vi "Operation Window.vi"(6 "Main UI Message Queue":refnum<queue>, 7 "UI State":T2, 8 "error in (no error)":errorcluster, 9 "Graph Notifier":refnum<notifier>, 10 "Message Queues":T21, 11 "Feed Module State Cluster in":T3={"Shared Variables"={"PID 1 Process Variable"="PID1-Mettler Toledo Scale 1", "PID 1 Output"="PID1-Mettler Toledo Scale 1", "PID 1 Setpoint"="PID1-Setpoint", "PID 1 Setpoint SV refnum"="ni.var.psp://localhost/Flow Module 1/PID1-Setpoint", "PID 1 Process Variable SV refnum"="ni.var.psp://localhost/Flow Module 1/PID1-Setpoint", "PID 1 Output SV refnum"="ni.var.psp://localhost/Flow Module 1/PID1-Setpoint"}, "Feed Module Config"={"GUID"="", "Drop Coords"={"Horizontal"=0, "Vertical"=0}, "Process Name"="", "Settings"={"Cycle Period"=500.0, "Ismatech"={"VISA resource name"="", "Simulated?"=TRUE, "Pump Number"=1.0, "Reverse?"=FALSE}, "Masterflex"={"VISA resource name"="", "Simulated?"=TRUE, "Pump Number"=1.0, "Reverse?"=FALSE}, "Mettler"={"VISA resource name"="", "Simulated?"=FALSE}, "Bronkhorst M13 Flow Meter"={"VISA resource name"="", "Simulated?"=TRUE}, "PID 2 Parameters"={"Input Device"=enum."Default", "Output Device"=enum."Default", "Setpoint"=0.0, "PID gains"={"proportional gain (Kc)"=1.0, "integral time (Ti, min)"=0.01, "derivative time (Td, min)"=0.0}}, "Manual Entry"=0.0, "Auto?"=TRUE, "output range"={"output high"=100.0, "output low"=0.0}, "Bronkhorst M14"={"VISA resource name"="", "Simulated?"=FALSE}, "Tacmina Settings"={"Analog DAQ Task"="", "Digital DAQ Task"=""}, "KNF SIMDOS Settings"={"VISA resource name"="", "Simulated?"=TRUE}, "ASIA Pump C"={"ASIA Pump #"=0, "channel"=0, "Simulated"=FALSE}, "VICI Settings"={"VISA resource name"="", "Simulated?"=TRUE, "Pump Letter"="", "Reverse?"=FALSE}, "FLOM Settings"={"VISA resource name"="", "Simulated?"=TRUE, "Pump Number"=0.0}, "SSI PR Settings"={"VISA resource name"="", "Simulated?"=FALSE}}, "Settings Load Count"=0, "OP Load Count"=0}} {"Feed Module Config"."Settings"."output range"."output low" min=0.0 max=100.0 format="%.2f"; "Feed Module Config"."Settings"."output range"."output high" format="%.2f"; "Feed Module Config"."Settings"."PID 2 Parameters"."PID gains"."derivative time (Td, min)" format="%.3f"; "Feed Module Config"."Settings"."PID 2 Parameters"."PID gains"."integral time (Ti, min)" format="%.3f"; "Feed Module Config"."Settings"."PID 2 Parameters"."PID gains"."proportional gain (Kc)" format="%.3f"; "Feed Module Config"."Settings"."ASIA Pump C"."channel" min=0 max=1 step=1; "Feed Module Config"."Settings"."Ismatech"."Pump Number" min=1.0 max=20.0 step=1.0; "Feed Module Config"."Settings"."Masterflex"."Pump Number" min=1.0 max=20.0 step=1.0}) -> (0 "error out":errorcluster, 2 "Need Update":bool, 3 "Feed Module State Cluster out":T3={"Shared Variables"={"PID 1 Process Variable"="PID1-Mettler Toledo Scale 1", "PID 1 Output"="PID1-Mettler Toledo Scale 1", "PID 1 Setpoint"="PID1-Setpoint", "PID 1 Setpoint SV refnum"="ni.var.psp://localhost/Flow Module 1/PID1-Setpoint", "PID 1 Process Variable SV refnum"="ni.var.psp://localhost/Flow Module 1/PID1-Setpoint", "PID 1 Output SV refnum"="ni.var.psp://localhost/Flow Module 1/PID1-Setpoint"}, "Feed Module Config"={"GUID"="", "Drop Coords"={"Horizontal"=0, "Vertical"=0}, "Process Name"="", "Settings"={"Cycle Period"=500.0, "Ismatech"={"VISA resource name"="", "Simulated?"=TRUE, "Pump Number"=1.0, "Reverse?"=FALSE}, "Masterflex"={"VISA resource name"="", "Simulated?"=TRUE, "Pump Number"=1.0, "Reverse?"=FALSE}, "Mettler"={"VISA resource name"="", "Simulated?"=FALSE}, "Bronkhorst M13 Flow Meter"={"VISA resource name"="", "Simulated?"=TRUE}, "PID 2 Parameters"={"Input Device"=enum."Default", "Output Device"=enum."Default", "Setpoint"=0.0, "PID gains"={"proportional gain (Kc)"=1.0, "integral time (Ti, min)"=0.01, "derivative time (Td, min)"=0.0}}, "Manual Entry"=0.0, "Auto?"=TRUE, "output range"={"output high"=100.0, "output low"=0.0}, "Bronkhorst M14"={"VISA resource name"="", "Simulated?"=FALSE}, "Tacmina Settings"={"Analog DAQ Task"="", "Digital DAQ Task"=""}, "KNF SIMDOS Settings"={"VISA resource name"="", "Simulated?"=TRUE}, "ASIA Pump C"={"ASIA Pump #"=0, "channel"=0, "Simulated"=FALSE}, "VICI Settings"={"VISA resource name"="", "Simulated?"=TRUE, "Pump Letter"="", "Reverse?"=FALSE}, "FLOM Settings"={"VISA resource name"="", "Simulated?"=TRUE, "Pump Number"=0.0}, "SSI PR Settings"={"VISA resource name"="", "Simulated?"=FALSE}}, "Settings Load Count"=0, "OP Load Count"=0}} {"Feed Module Config"."Settings"."output range"."output low" min=0.0 max=100.0 format="%.2f"; "Feed Module Config"."Settings"."output range"."output high" format="%.2f"; "Feed Module Config"."Settings"."PID 2 Parameters"."PID gains"."derivative time (Td, min)" format="%.3f"; "Feed Module Config"."Settings"."PID 2 Parameters"."PID gains"."integral time (Ti, min)" format="%.3f"; "Feed Module Config"."Settings"."PID 2 Parameters"."PID gains"."proportional gain (Kc)" format="%.3f"; "Feed Module Config"."Settings"."ASIA Pump C"."channel" min=0 max=1 step=1; "Feed Module Config"."Settings"."Ismatech"."Pump Number" min=1.0 max=20.0 step=1.0; "Feed Module Config"."Settings"."Masterflex"."Pump Number" min=1.0 max=20.0 step=1.0})   [LabVIEW 2018, in "Feed Module.lvlib"]
uses:
  Feed Module/Feed Module.lvlib
  Feed Module/Controls/Feed Message Queues.ctl
  support/Message Queue/Message Cluster.ctl
  Feed Module/Controls/Feed Module State Cluster.ctl
  Feed Module/Controls/Feed Module Shared Variable Cluster.ctl
  Feed Module/Controls/Feed Module Config Cluster.ctl
  <vilib>/Utility/miscctls.llb/LVPoint32TypeDef.ctl
  Feed Module/Controls/Feed Module Settings Cluster.ctl
  Ismatec ISM 831C/Controls/Ismatech Settings Cluster.ctl
  Masterflex 7550-30/Controls/Settings Cluster.ctl
  Mettler Toledo/Controls/Settings Cluster.ctl
  Bronkhorst M13 Flow Meter/Settings Cluster.ctl
  Measure Instrument/PID 2 Parameters Cluster.ctl
  Measure Instrument/PID Input Enum.ctl
  Measure Instrument/PID 2 Output Enum.ctl
  Tacmina QI/Tacmina QI DAQ Setting.ctl
  KNF Pump/Settings Cluster plus SIMDOS.ctl
  ASIA Pump/Pump Settings.ctl
  VICI M50 Party Mode/Settings Cluster.ctl
  FLOM Pump/Settings Cluster.ctl
  SSI PR Class/SSI PR Settings Cluster.ctl
  controls/UI State.ctl
  Config Module/Controls/OP Window Display.ctl
  support/Message Queue/Enqueue Message (Single).vi
  support/Message Queue/Message Queue.lvlib
  support/Support Library.lvlib
  Settings/Settings Dialog.vi
  Settings/Settings.lvlib
  Ismatec ISM 831C/Ismatec ISM 831C.lvlib
  Masterflex 7550-30/Masterflex 7550-30.lvlib
  Mettler Toledo/Mettler Toledo.lvlib
  Bronkhorst M13 Flow Meter/Bronkhorst M13 Flow Meter.lvlib
  Tacmina QI/Tacmina QI.lvlib
  KNF Pump/KNF SIMDOS.lvlib
  ASIA Pump.lvlib
  VICI M50 Party Mode/VICI M6 M50 Party Mode.lvlib
  FLOM Pump/FLOM Pump.lvlib
  SSI PR Class/SSI PR Pump.lvlib
panel:
  out "Start button status":T1(ring)
  out "Started":bool
  out "Updated":bool
  out "Flow":dbl caption="gm/min" format="%.2f"
  out "Data":waveform(dbl)[](graph)
  in  "Auto?":bool=TRUE
  in  "Manual Entry":dbl step=0.1 format="%#_6f"
  in  "Setpoint":dbl
  in  "Cancel Button":bool
  in  "OK Button":bool
  in  "Start":bool
  in  "Settings":bool
  in  "Stop":bool
  # "Output Instruments"
  # "Input Instruments"
  # "Output Instruments"
  # "Input Instruments"
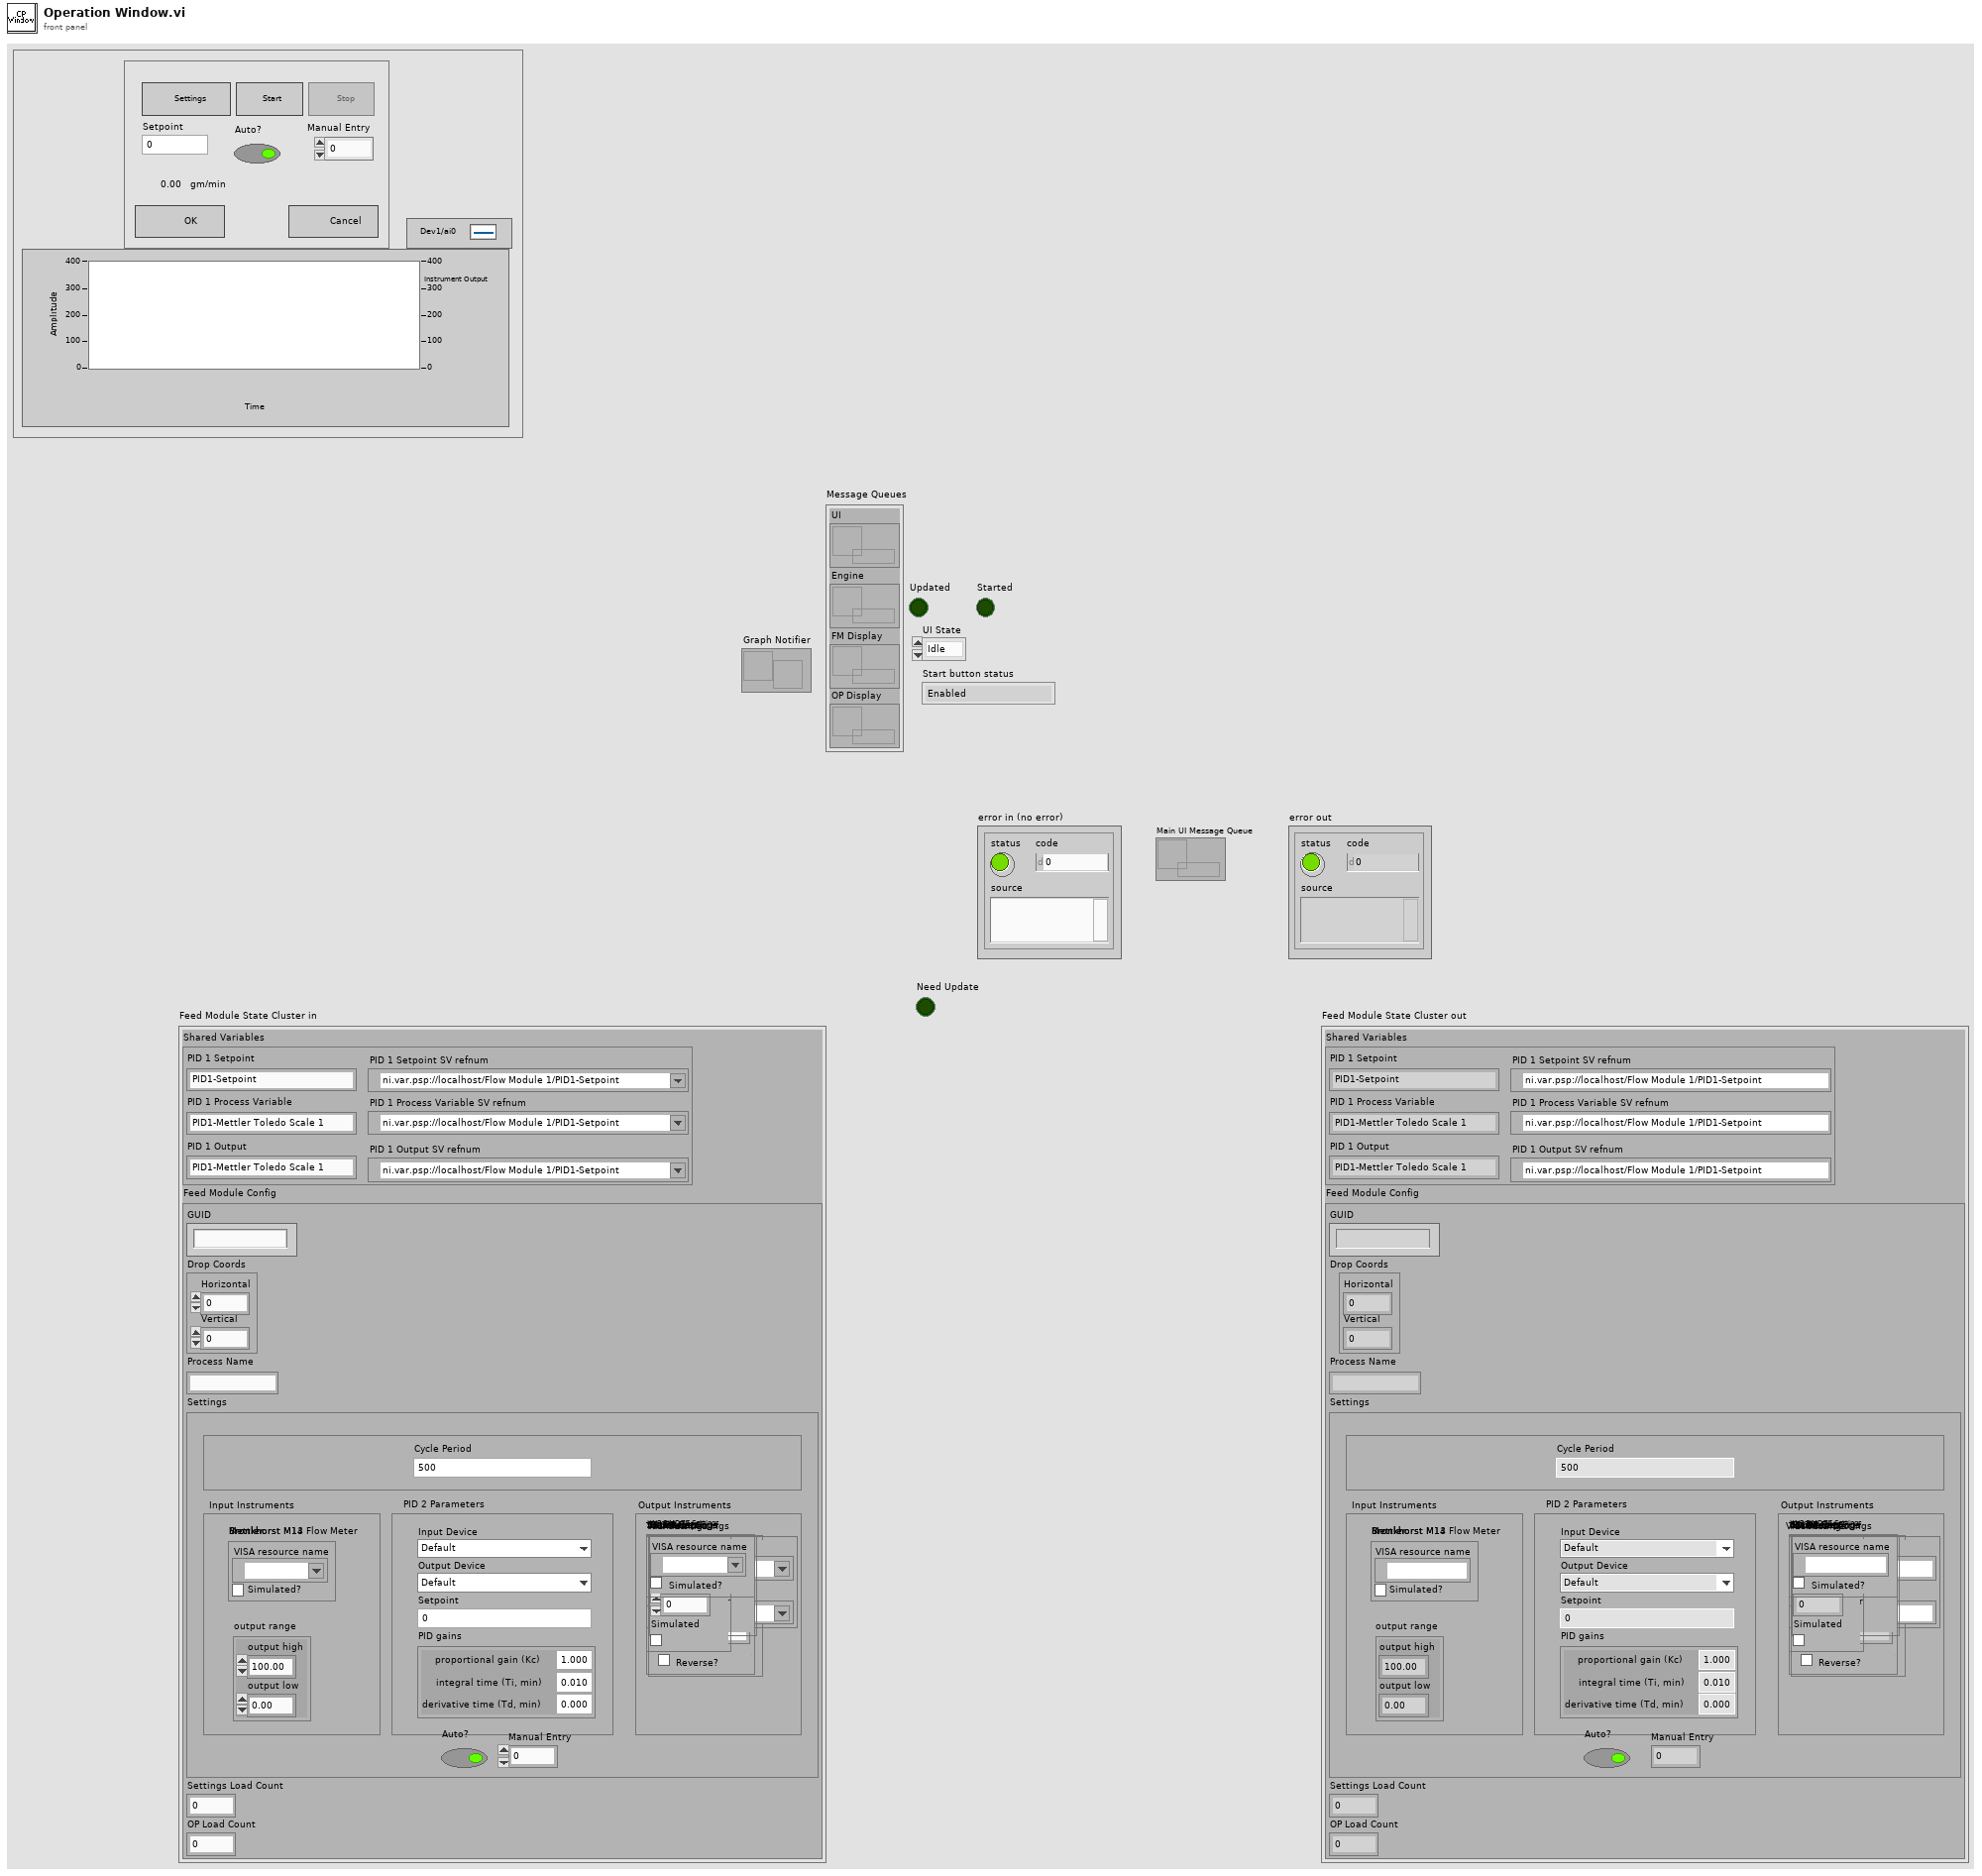
[diagram p1: front panel]
types:
  T1 = enum8{"Enabled", "Disabled", "Disabled and Grayed Out"}
  T2 = typedef "UI State.ctl" = enum16{"Idle", "Acquiring and Logging", "Waiting for Exit", "Waiting for Exit (Acq Stopped)", "Waiting for Exit (Log Stopped)", "Waiting for Stop", "Waiting for Stop (Acq Stopped)", "Waiting for Stop (Log Stopped)"}
  T3 = typedef "Feed Module.lvlib/Feed Module State Cluster.ctl" = cluster{"Shared Variables":T4, "Feed Module Config":T5}
  T4 = typedef "Feed Module.lvlib/Feed Module Shared Variable Cluster.ctl" = cluster{"PID 1 Process Variable":string, "PID 1 Output":string, "PID 1 Setpoint":string, "PID 1 Setpoint SV refnum":refnum<k21>, "PID 1 Process Variable SV refnum":refnum<k21>, "PID 1 Output SV refnum":refnum<k21>}
  T5 = typedef "Feed Module.lvlib/Feed Module Config Cluster.ctl" = cluster{"GUID":string, "Drop Coords":T6, "Process Name":string, "Settings":T7, "Settings Load Count":i32, "OP Load Count":i32}
  T6 = typedef "LVPoint32TypeDef.ctl" = cluster{"Horizontal":i32, "Vertical":i32}
  T7 = typedef "Feed Module.lvlib/Feed Module Settings Cluster.ctl" = cluster{"Cycle Period":dbl, "Ismatech":T8, "Masterflex":T9, "Mettler":T10, "Bronkhorst M13 Flow Meter":T11, "PID 2 Parameters":T12, "Manual Entry":dbl, "Auto?":bool, "output range":cluster{"output high":dbl, "output low":dbl}, "Bronkhorst M14":T10, "Tacmina Settings":T15, "KNF SIMDOS Settings":T16, "ASIA Pump C":T17, "VICI Settings":T18, "FLOM Settings":T19, "SSI PR Settings":T20}
  T8 = typedef "Ismatec ISM 831C.lvlib/Ismatech Settings Cluster.ctl" = cluster{"VISA resource name":refnum<visa-resource-name>, "Simulated?":bool, "Pump Number":dbl, "Reverse?":bool}
  T9 = typedef "Masterflex 7550-30.lvlib/Settings Cluster.ctl" = cluster{"VISA resource name":refnum<visa-resource-name>, "Simulated?":bool, "Pump Number":dbl, "Reverse?":bool}
  T10 = typedef "Mettler Toledo.lvlib/Settings Cluster.ctl" = cluster{"VISA resource name":refnum<visa-resource-name>, "Simulated?":bool}
  T11 = typedef "Bronkhorst M13 Flow Meter.lvlib/Settings Cluster.ctl" = cluster{"VISA resource name":refnum<visa-resource-name>, "Simulated?":bool}
  T12 = typedef "PID 2 Parameters Cluster.ctl" = cluster{"Input Device":T13, "Output Device":T14, "Setpoint":dbl, "PID gains":cluster{"proportional gain (Kc)":dbl, "integral time (Ti, min)":dbl, "derivative time (Td, min)":dbl}}
  T13 = typedef "PID Input Enum.ctl" = enum16{"Default", "Bronkhorst M13", "Bronkhorst M14", "Scale Rate of Change"}
  T14 = typedef "PID 2 Output Enum.ctl" = enum16{"Default", "Ismatec ISM 831C", "Masterflex 7550-30", "VICI", "Tacmina QI", "KNF SIMDOS", "ASIA Type C", "FLOM UI-22-11", "SSI PR"}
  T15 = typedef "Tacmina QI.lvlib/Tacmina QI DAQ Setting.ctl" = cluster{"Analog DAQ Task":refnum<k21>, "Digital DAQ Task":refnum<k21>}
  T16 = typedef "KNF SIMDOS.lvlib/Settings Cluster plus SIMDOS.ctl" = cluster{"VISA resource name":refnum<visa-resource-name>, "Simulated?":bool}
  T17 = typedef "ASIA Pump.lvlib/Pump Settings.ctl" = cluster{"ASIA Pump #":i32, "channel":i32, "Simulated":bool}
  T18 = typedef "VICI M6 M50 Party Mode.lvlib/Settings Cluster.ctl" = cluster{"VISA resource name":refnum<visa-resource-name>, "Simulated?":bool, "Pump Letter":string, "Reverse?":bool}
  T19 = typedef "FLOM Pump.lvlib/Settings Cluster.ctl" = cluster{"VISA resource name":refnum<visa-resource-name>, "Simulated?":bool, "Pump Number":dbl}
  T20 = typedef "SSI PR Pump.lvlib/SSI PR Settings Cluster.ctl" = cluster{"VISA resource name":refnum<visa-resource-name>, "Simulated?":bool}
  T21 = typedef "Feed Module.lvlib/Feed Message Queues.ctl" = cluster{"UI":refnum<queue>, "Engine":refnum<queue>, "FM Display":refnum<queue>, "OP Display":refnum<queue>}
  T22 = typedef "Feed Module.lvlib/OP Window Display.ctl" = cluster{"Flow":dbl, "Manual":dbl, "Pump Status":u16}
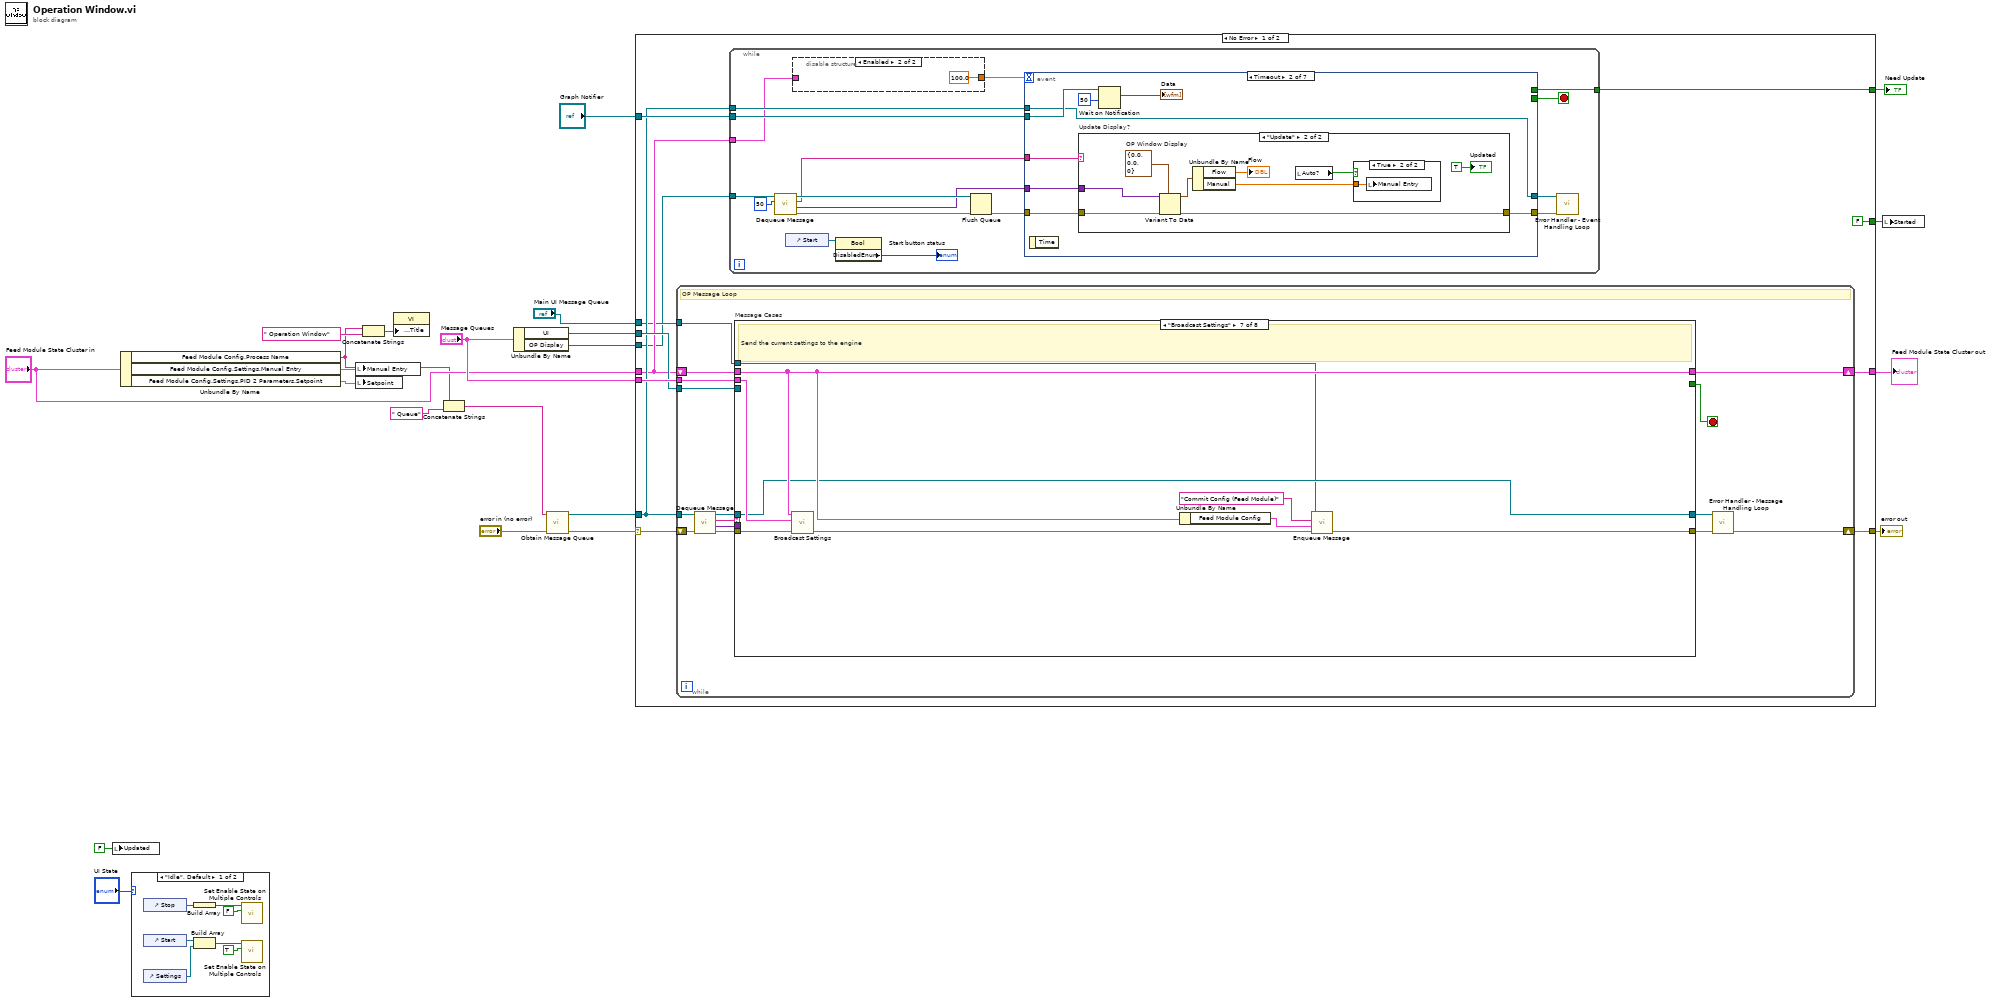
[diagram p0: block diagram]
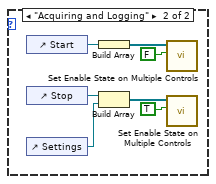
[diagram p2: hidden frame]
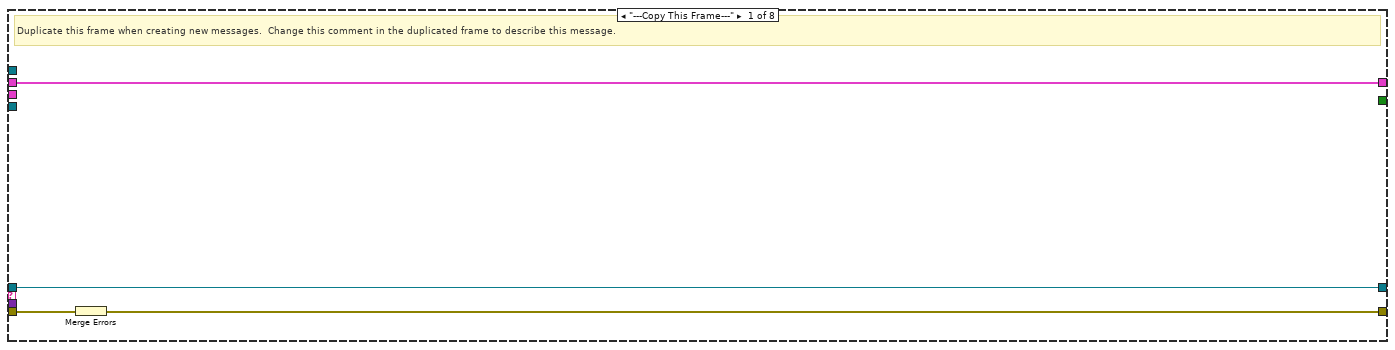
[diagram p3: hidden frame]
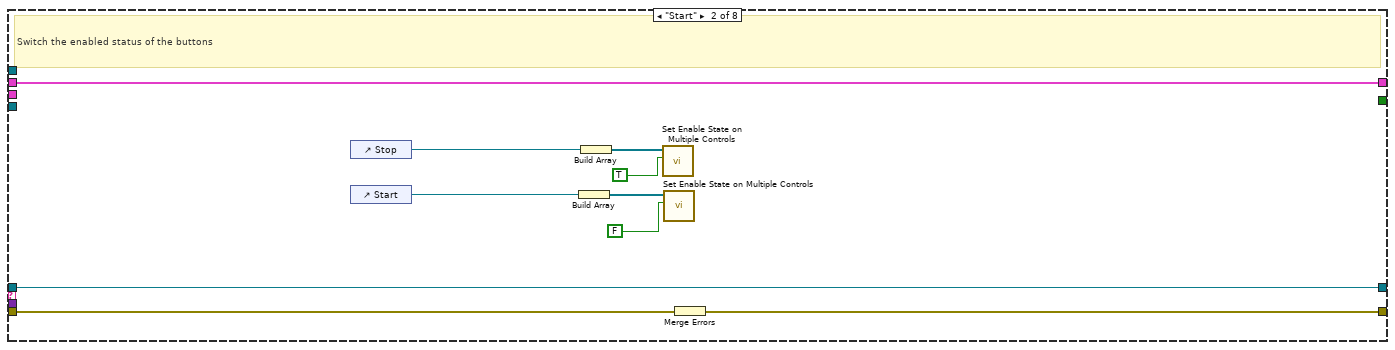
[diagram p4: hidden frame]
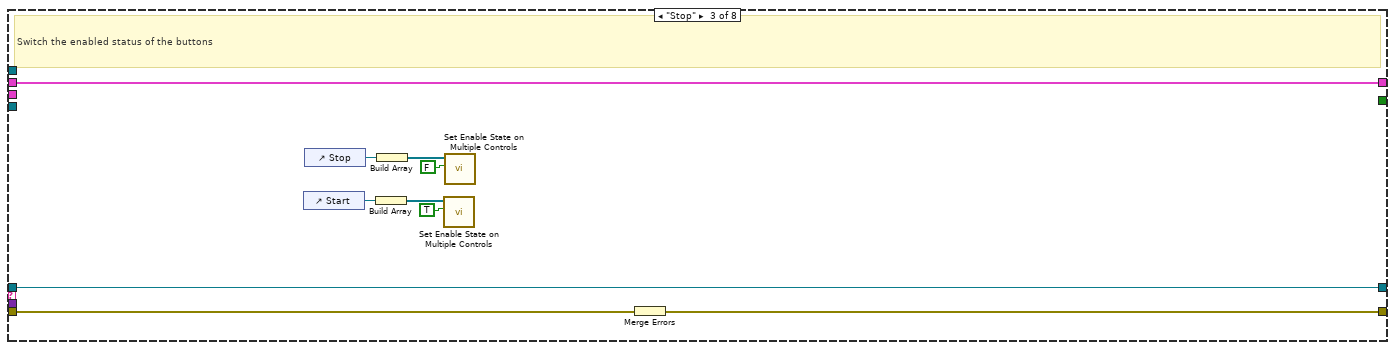
[diagram p5: hidden frame]
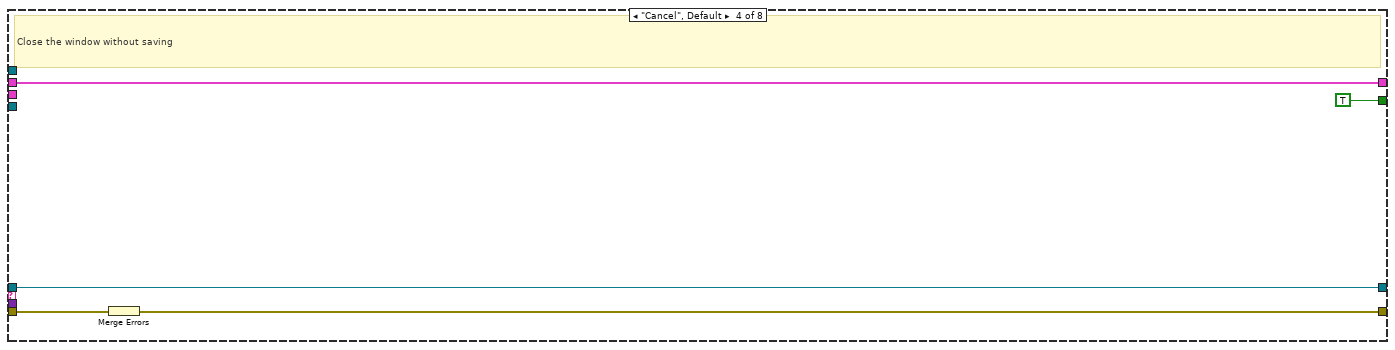
[diagram p6: hidden frame]
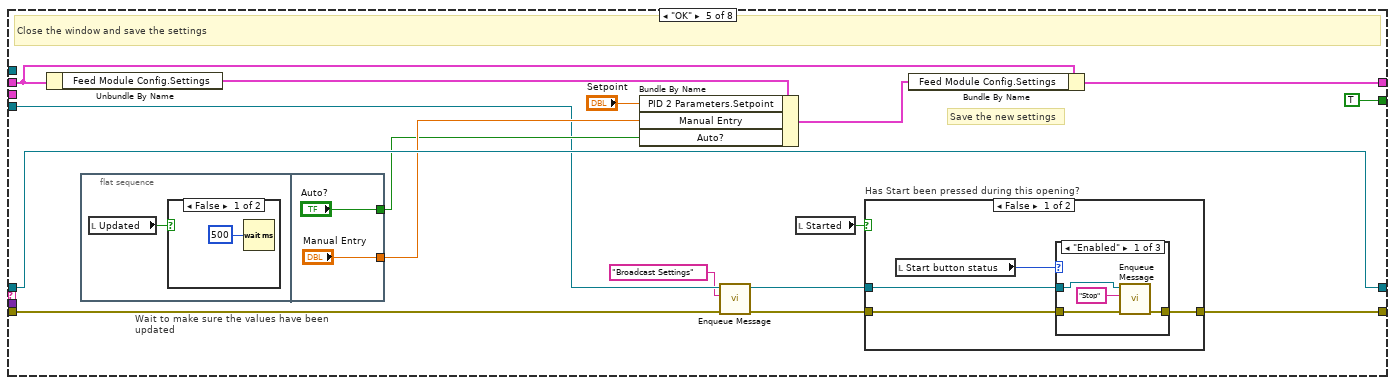
[diagram p7: hidden frame]
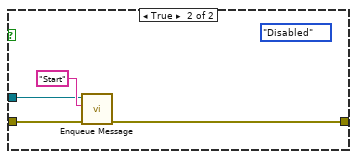
[diagram p10: hidden frame]
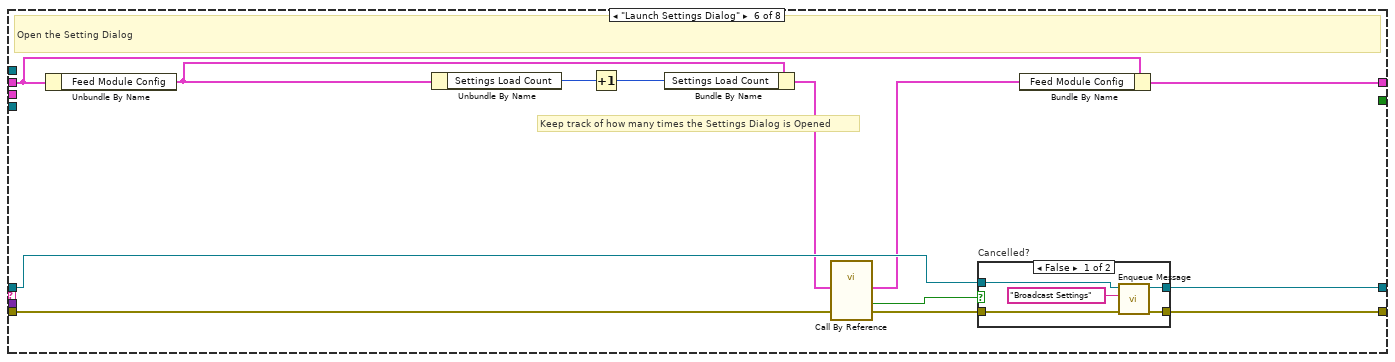
[diagram p12: hidden frame]
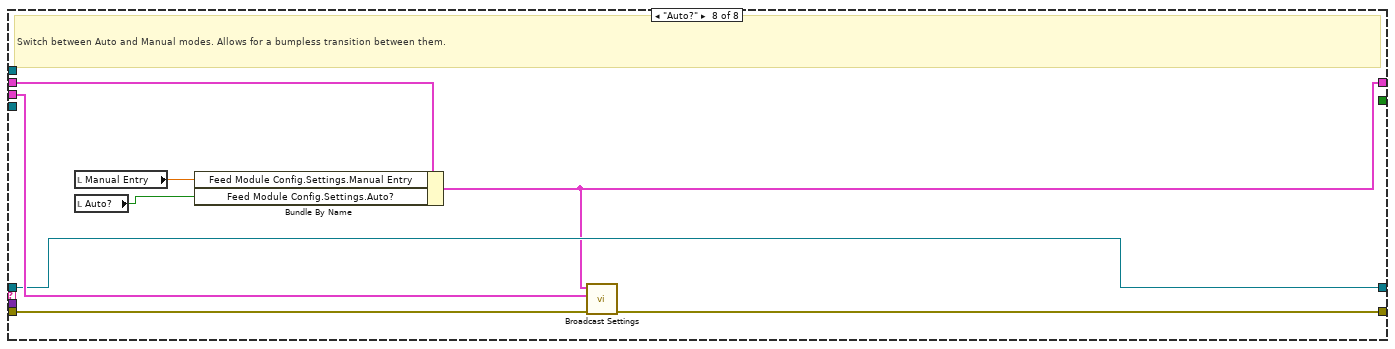
[diagram p14: hidden frame]
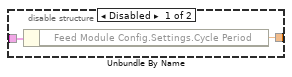
[diagram p15: hidden frame]
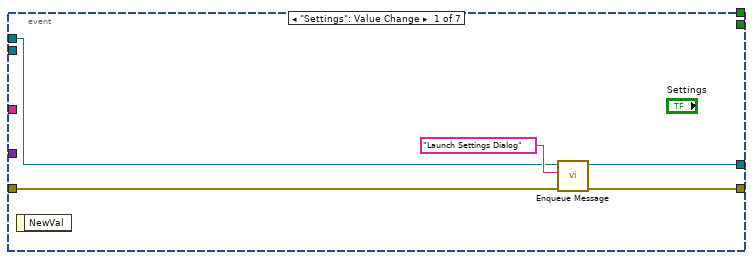
[diagram p16: hidden frame]
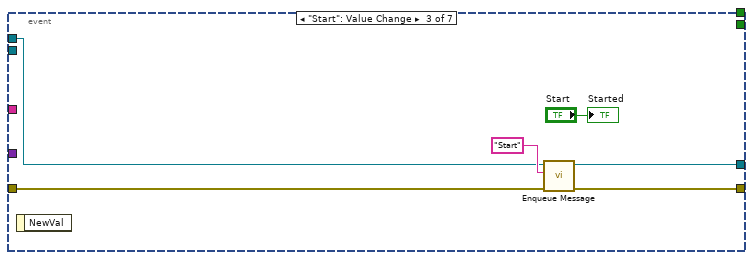
[diagram p19: hidden frame]
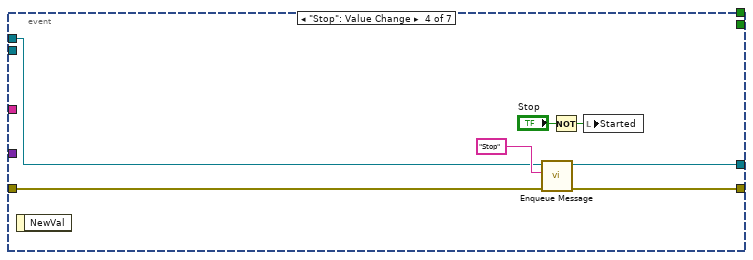
[diagram p20: hidden frame]
diagram:
  n1 = local write "Updated"(FALSE ("Boolean")) -> ()
  n2 = Unbundle By Name("Feed Module State Cluster in") -> ("Feed Module Config.Process Name"=w6:string, "Feed Module Config.Settings.Manual Entry"=w12:dbl, "Feed Module Config.Settings.PID 2 Parameters.Setpoint"=w10:dbl)
  n3 = case shown="\"Idle\", Default" "UI State" {
    frame "Idle", Default {
      n4 = control-ref of="Stop"() -> (w23:refnum<vi>)
      n5 = control-ref of="Start"() -> (w25:refnum<vi>)
      n6 = control-ref of="Settings"() -> (w24:refnum<vi>)
      n7 = Build Array(w23) -> (w27:refnum<vi>[])
      n8 = Build Array(w25, w24) -> (w28:refnum<vi>[])
      n9 = call "Set Enable State on Multiple Controls.vi"("Enable?"=FALSE, "Controls"=w27) -> ()  [unwired: 10 in]
      n10 = call "Set Enable State on Multiple Controls.vi"("Enable?"=TRUE, "Controls"=w28) -> ()  [unwired: 10 in]
    }
    frame "Acquiring and Logging" {
      n11 = control-ref of="Start"() -> (w32:refnum<vi>)
      n12 = control-ref of="Stop"() -> (w31:refnum<vi>)
      n13 = control-ref of="Settings"() -> (w30:refnum<vi>)
      n14 = Build Array(w32) -> (w35:refnum<vi>[])
      n15 = Build Array(w31, w30) -> (w34:refnum<vi>[])
      n16 = call "Set Enable State on Multiple Controls.vi"("Enable?"=FALSE, "Controls"=w35) -> ()  [unwired: 10 in]
      n17 = call "Set Enable State on Multiple Controls.vi"("Enable?"=TRUE, "Controls"=w34) -> ()  [unwired: 10 in]
    }
  }
  n18 = local write "Manual Entry"(w12) -> ()
  n19 = local write "Setpoint"(w10) -> ()
  n20 = Concatenate Strings(w6, " Operation Window" ("string")) -> (w5:string)
  n21 = property class="VI"("Front Panel.Title"=w5) -> ()  [unwired: 2 in, 2 out]
  n22 = Concatenate Strings(w6, " Queue" ("string")) -> (w9:string)
  n23 = Unbundle By Name("Message Queues") -> ("UI"=w16:refnum<queue>, "OP Display"=w13:refnum<queue>)
  n24 = call "Obtain Message Queue.vi"("error in (no error)"="error in (no error)", "name (unnamed)"=w9) -> ("error out"=w2:errorcluster, "Message Queue"=w19:refnum<queue>)  [unwired: 8 in]
  n25 = case shown="No Error" w2 {
    selector: w2 -> [w37 w243]
    tunnel: [w41 w243] -> w22
    tunnel: [w48 FALSE] -> w21
    tunnel: w19 -> [w43 _]
    tunnel: "Feed Module State Cluster in" -> [w42 w241]
    tunnel: [w47 w241] -> w14
    tunnel: "Message Queues" -> [w46 _]
    tunnel: "Graph Notifier" -> [w45 _]
    tunnel: w16 -> [w44 _]
    tunnel: "Main UI Message Queue" -> [w40 _]
    tunnel: w13 -> [w39 _]
    tunnel: [FALSE FALSE] -> w3
    frame No Error {
      n26 = while {
        shift-right: [w52] -> w41
        shift-left: w37 -> [w55]
        tunnel: w43 -> [w54]
        tunnel: w46 -> [w56]
        shift-right: [w57] -> w47
        shift-left: w42 -> [w53]
        tunnel: w44 -> [w51]
        tunnel: w40 -> [w49]
        stop <- w58 stop-if-true
        # "OP Message Loop"
        n27 = call "Dequeue Message.vi"("error in (no error)"=w55, "Message Queue"=w54) -> ("error out"=w59:errorcluster, "Message Data"=w62:variant, "Message"=w63:string, "dup Message Queue"=w60:refnum<queue>)  [unwired: 6 in]
        n28 = case "Message Cases" shown="\"Broadcast Settings\"" w63 {
          tunnel: w60 -> [w64 w68 w78 w88 w106 w135 w152 w161]
          tunnel: w59 -> [w67 w77 w87 w92 w98 w128 w154 w162]
          tunnel: [w66 w76 w86 w91 w96 w137 w151 w156] -> w61
          tunnel: w62 -> [_ _ _ _ _ _ _ _]
          tunnel: [_ _ _ TRUE TRUE _ _ _] -> w58
          tunnel: w53 -> [w65 w69 w85 w89 w102 w136 w153 w158]
          tunnel: [w65 w69 w85 w89 w105 w130 w153 w157] -> w57
          tunnel: w56 -> [_ _ _ _ _ _ w155 w163]
          tunnel: w51 -> [_ _ _ _ w99 _ _ _]
          tunnel: [w64 w68 w78 w88 w106 w134 w152 w161] -> w50
          tunnel: w49 -> [_ _ _ _ _ _ w148 _]
          frame "---Copy This Frame---" {
            # "Duplicate this frame when creating new messages.  Change this comment in the duplicated frame to describe this message."
            n29 = Merge Errors(w67) -> (w66:errorcluster)
          }
          frame "Start" {
            # "Switch the enabled status of the buttons"
            n30 = control-ref of="Stop"() -> (w74:refnum<vi>)
            n31 = control-ref of="Start"() -> (w75:refnum<vi>)
            n32 = Build Array(w75) -> (w72:refnum<vi>[])
            n33 = Build Array(w74) -> (w73:refnum<vi>[])
            n34 = call "Set Enable State on Multiple Controls.vi"("Enable?"=TRUE, "Controls"=w73) -> ()  [unwired: 10 in]
            n35 = call "Set Enable State on Multiple Controls.vi"("Enable?"=FALSE, "Controls"=w72) -> ()  [unwired: 10 in]
            n36 = Merge Errors(w77) -> (w76:errorcluster)
          }
          frame "Stop" {
            # "Switch the enabled status of the buttons"
            n37 = control-ref of="Start"() -> (w84:refnum<vi>)
            n38 = control-ref of="Stop"() -> (w81:refnum<vi>)
            n39 = Build Array(w84) -> (w83:refnum<vi>[])
            n40 = Build Array(w81) -> (w80:refnum<vi>[])
            n41 = call "Set Enable State on Multiple Controls.vi"("Enable?"=TRUE, "Controls"=w83) -> ()  [unwired: 10 in]
            n42 = call "Set Enable State on Multiple Controls.vi"("Enable?"=FALSE, "Controls"=w80) -> ()  [unwired: 10 in]
            n43 = Merge Errors(w87) -> (w86:errorcluster)
          }
          frame "Cancel", Default {
            # "Close the window without saving"
            n44 = Merge Errors(w92) -> (w91:errorcluster)
          }
          frame "OK" {
            # "Save the new settings"
            # "Close the window and save the settings"
            n45 = Unbundle By Name(w102) -> ("Feed Module Config.Settings"=w103:T7)
            n46 = flat-sequence "Wait to make sure the values have been updated" {
              tunnel: ["Manual Entry"] -> w101
              tunnel: ["Auto?"] -> w100
              frame #0 {
                n47 = local read "Updated"() -> (w123:bool)
                n48 = case shown="False" w123 {
                  frame False {
                    n49 = Wait (ms)(milliseconds to wait=u32 500) -> ()  [unwired: 1 out]
                  }
                  frame True {
                  }
                }
              }
              frame #1 {
              }
            }
            n50 = Bundle By Name(cluster=w103, "PID 2 Parameters.Setpoint"="Setpoint", "Manual Entry"=w101, "Auto?"=w100) -> (w104:T7)
            n51 = call-poly "Enqueue Message.vi"("error in (no error)"=w98, "Message"="Broadcast Settings", "Message Queue"=w99) -> ("error out"=w93:errorcluster, "dup Message Queue"=w94:refnum<queue>)  [unwired: 7 in]
            n52 = local read "Started"() -> (w97:bool)
            n53 = case "Has Start been pressed during this opening?" shown="False" w97 {
              tunnel: w94 -> [w110 w121]
              tunnel: w93 -> [w111 w120]
              tunnel: [w112 w119] -> w96
              frame False {
                n54 = local read "Start button status"() -> (w109:T1)
                n55 = case shown="\"Enabled\"" w109 {
                  tunnel: [w115 w117 w118] -> w112
                  tunnel: w111 -> [w114 w117 w118]
                  tunnel: w110 -> [w113 _ _]
                  frame "Enabled" {
                    n56 = call-poly "Enqueue Message.vi"("error in (no error)"=w114, "Message"="Stop", "Message Queue"=w113) -> ("error out"=w115:errorcluster)  [unwired: 7 in, 1 out]
                  }
                  frame "Disabled" {
                  }
                  frame "Disabled and Grayed Out" {
                  }
                }
              }
              frame True {
                (unwired) T1."Disabled" ("DisabledEnum")
                n57 = call-poly "Enqueue Message.vi"("error in (no error)"=w120, "Message"="Start", "Message Queue"=w121) -> ("error out"=w119:errorcluster)  [unwired: 7 in, 1 out]
              }
            }
            n58 = Bundle By Name(cluster=w102, "Feed Module Config.Settings"=w104) -> (w105:T3)
          }
          frame "Launch Settings Dialog" {
            # "Keep track of how many times the Settings Dialog is Opened"
            # "Open the Setting Dialog"
            n59 = Unbundle By Name(w136) -> ("Feed Module Config"=w132:T5)
            n60 = Unbundle By Name(w132) -> ("Settings Load Count"=w131:i32)
            n61 = Increment(x=w131) -> (x+1=w133:i32)
            n62 = Bundle By Name(cluster=w132, "Settings Load Count"=w133) -> (w127:T5)
            n63 = call-by-ref "?"("error in (no error)"=w128, "Feed Module Config in"=w127) -> ("error out"=w138:errorcluster, "Cancelled?"=w139:bool, "Feed Module Config out"=w129:T5)  [unwired: 8 in, 3 out]
            n64 = case "Cancelled?" shown="False" w139 {
              tunnel: [w144 w146] -> w137
              tunnel: w138 -> [w142 w146]
              tunnel: w135 -> [w141 w145]
              tunnel: [w140 w145] -> w134
              frame False {
                n65 = call-poly "Enqueue Message.vi"("error in (no error)"=w142, "Message"="Broadcast Settings", "Message Queue"=w141) -> ("error out"=w144:errorcluster, "dup Message Queue"=w140:refnum<queue>)  [unwired: 7 in]
              }
              frame True {
              }
            }
            n66 = Bundle By Name(cluster=w136, "Feed Module Config"=w129) -> (w130:T3)
          }
          frame "Broadcast Settings" {
            # "Send the current settings to the engine"
            n67 = call "Broadcast Settings.vi"("error in (no error)"=w154, "Message Queues"=w155, "Feed Module State Cluster in"=w153) -> ("error out"=w150:errorcluster)  [unwired: 8 in]
            n68 = Unbundle By Name(w153) -> ("Feed Module Config"=w149:T5)
            n69 = call-poly "Enqueue Message.vi"("error in (no error)"=w150, "Message Data"=w149, "Message"="Commit Config (Feed Module)", "Message Queue"=w148) -> ("error out"=w151:errorcluster)  [unwired: 6 in, 1 out]
          }
          frame "Auto?" {
            # "Switch between Auto and Manual modes. Allows for a bumpless transition between them."
            n70 = local read "Manual Entry"() -> (w160:dbl)
            n71 = local read "Auto?"() -> (w159:bool)
            n72 = Bundle By Name(cluster=w158, "Feed Module Config.Settings.Manual Entry"=w160, "Feed Module Config.Settings.Auto?"=w159) -> (w157:T3)
            n73 = call "Broadcast Settings.vi"("error in (no error)"=w162, "Message Queues"=w163, "Feed Module State Cluster in"=w157) -> ("error out"=w156:errorcluster)  [unwired: 8 in]
          }
        }
        n74 = call "Error Handler - Message Handling Loop.vi"("error in (no error)"=w61, "Message Queue"=w50) -> ("dup error in"=w52:errorcluster)  [unwired: 8 in, 1 out]
      }
      n75 = while {
        tunnel: [w177] -> w48
        tunnel: w43 -> [w176]
        tunnel: w45 -> [w175]
        tunnel: w42 -> [w173]
        tunnel: w39 -> [w172]
        stop <- w178 stop-if-true
        n76 = call "Dequeue Message.vi"("timeout in ms (-1)"=50, "Message Queue"=w172) -> ("error out"=w170:errorcluster, "Message Data"=w167:variant, "Message"=w168:string, "dup Message Queue"=w169:refnum<queue>)  [unwired: 6 in]
        n77 = control-ref of="Start"() -> (w165:refnum<vi>)
        n78 = disable-structure shown="Enabled" {
          disable-tunnel: [w182 100.0 ("Cycle Period")] -> w174
          disable-tunnel: w173 -> [w181 _]
          frame Disabled {
            n79 = Unbundle By Name(w181) -> ("Feed Module Config.Settings.Cycle Period"=w182:dbl)
          }
          frame Enabled {
          }
        }
        n80 = property class="Bool"(reference=w165) -> ("DisabledEnum"=→"Start button status":T1)  [unwired: 1 in, 2 out]
        n81 = Flush Queue(queue=w169, error in (no error)=w170) -> (error out=w166:errorcluster)  [unwired: 2 out]
        n82 = event shown="[1] Timeout" {
          selector: _ -> [_ _ _ _ _ _ _]
          dyn-events: _ -> [_ _ _ _ _ _ _]
          timeout: w174 -> [_ _ _ _ _ _ _]
          tunnel: [w187 w189 w210 w218 w223 w230 w238] -> w180
          tunnel: [w186 w190 w211 w217 w222 w229 w237] -> w179
          tunnel: [_ _ _ _ _ TRUE ("Priority Message? (F)") w236] -> w178
          tunnel: [_ _ _ _ _ FALSE ("Priority Message? (F)") w236] -> w177
          tunnel: w176 -> [w185 w189 w212 w219 w224 w227 w235]
          tunnel: w175 -> [_ w195 _ _ _ _ _]
          tunnel: w168 -> [_ w193 _ _ _ _ _]
          tunnel: w167 -> [_ w192 _ _ _ _ _]
          tunnel: w166 -> [w184 w191 w208 w214 w221 w226 w234]
          event "Settings": Value Change {
            n83 = event-data() -> ()  [unwired: 1 in, 1 out]
            n84 = call-poly "Enqueue Message.vi"("error in (no error)"=w184, "Message"="Launch Settings Dialog", "Message Queue"=w185) -> ("error out"=w186:errorcluster, "dup Message Queue"=w187:refnum<queue>)  [unwired: 7 in]
          }
          event Timeout {
            n85 = event-data() -> ()  [unwired: 1 in, 1 out]
            n86 = case "Update Display?" shown="\"Update\"" w193 {
              tunnel: w192 -> [_ w206]
              tunnel: w191 -> [w197 w199]
              tunnel: [w197 w198] -> w190
              frame "False", Default {
              }
              frame "Update" {
                w205 = T22 {"Flow"=0.0, "Manual"=0.0, "Pump Status"=0}  # OP Window Display
                n87 = Variant To Data(error in=w199, type=w205, Variant=w206) -> (data=w204:T22, error out=w198:errorcluster)
                n88 = Unbundle By Name(w204) -> ("Flow"=→"Flow":dbl, "Manual"=w202:dbl)
                n89 = local read "Auto?"() -> (w201:bool)
                n90 = case shown="True" w201 {
                  tunnel: w202 -> [_ w207]
                  frame False {
                  }
                  frame True {
                    n91 = local write "Manual Entry"(w207) -> ()
                  }
                }
                "Updated" <- TRUE ("Boolean")
              }
            }
            n92 = Wait on Notification(notifier=w195, timeout in ms (-1)=50) -> (notification=→"Data":waveform(dbl)[])  [unwired: 2 in, 3 out]
          }
          event "Start": Value Change {
            n93 = event-data() -> ()  [unwired: 1 in, 1 out]
            n94 = call-poly "Enqueue Message.vi"("error in (no error)"=w208, "Message"="Start", "Message Queue"=w212) -> ("error out"=w211:errorcluster, "dup Message Queue"=w210:refnum<queue>)  [unwired: 7 in]
            "Started" <- "Start"
          }
          event "Stop": Value Change {
            n95 = event-data() -> ()  [unwired: 1 in, 1 out]
            n96 = call-poly "Enqueue Message.vi"("error in (no error)"=w214, "Message"="Stop", "Message Queue"=w219) -> ("error out"=w217:errorcluster, "dup Message Queue"=w218:refnum<queue>)  [unwired: 7 in]
            n97 = Not(x="Stop") -> (.not. x?=w215:bool)
            n98 = local write "Started"(w215) -> ()
          }
          event "Auto?": Value Change {
            n99 = event-data() -> ()  [unwired: 1 in, 1 out]
            n100 = call-poly "Enqueue Message.vi"("error in (no error)"=w221, "Message"="Auto?", "Message Queue"=w224) -> ("error out"=w222:errorcluster, "dup Message Queue"=w223:refnum<queue>)  [unwired: 7 in]
          }
          event "Cancel Button": Value Change {
            n101 = event-data() -> ()  [unwired: 1 in, 1 out]
            n102 = call-poly "Enqueue Message.vi"("Priority Message? (F)"=TRUE, "error in (no error)"=w226, "Message"="Cancel", "Message Queue"=w227) -> ("error out"=w229:errorcluster, "dup Message Queue"=w230:refnum<queue>)  [unwired: 6 in]
          }
          event "OK Button": Value Change {
            w236 = TRUE
            n103 = event-data() -> ()  [unwired: 1 in, 1 out]
            n104 = call-poly "Enqueue Message.vi"("error in (no error)"=w234, "Message"="OK", "Message Queue"=w235) -> ("error out"=w237:errorcluster, "dup Message Queue"=w238:refnum<queue>)  [unwired: 7 in]
          }
        }
        n105 = call "Error Handler - Event Handling Loop.vi"("error in (no error)"=w179, "Message Queue"=w180) -> ()  [unwired: 8 in, 2 out]
      }
    }
    frame Error {
    }
  }
  "error out" <- w22
  "Need Update" <- w21
  "Feed Module State Cluster out" <- w14
  n106 = local write "Started"(w3) -> ()
